vi "GetEdgeMenu.vi"(0 "reference":refnum<class "StateTransitionEdge.lvclass">, 5 "error in (no error)":errorcluster) -> (14 "reference out":refnum<class "StateTransitionEdge.lvclass">, 15 "MenuOptions":string[](array[string]), 19 "error out":errorcluster)   [LabVIEW 2016, in "StateTransitionEdge.lvclass"]
doc: "GetEdgeMenu"
uses:
  <resource>/Framework/Providers/Open_GDS/UML/StateTransitionEdge_class/StateTransitionEdge.lvclass
  C:/Program Files (x86)/National Instruments/LabVIEW 2016/resource/Framework/Providers/Open_GDS/UML/ClassRelationshipEdge_class/ClassRelationshipEdge.lvclass
  <resource>/Framework/Providers/Open_GDS/UML/ClassRelationshipEdge_class/ClassRelationshipEdge.lvclass
  <resource>/Framework/Providers/Open_GDS/UML/BentStyle_class/BentStyle.lvclass
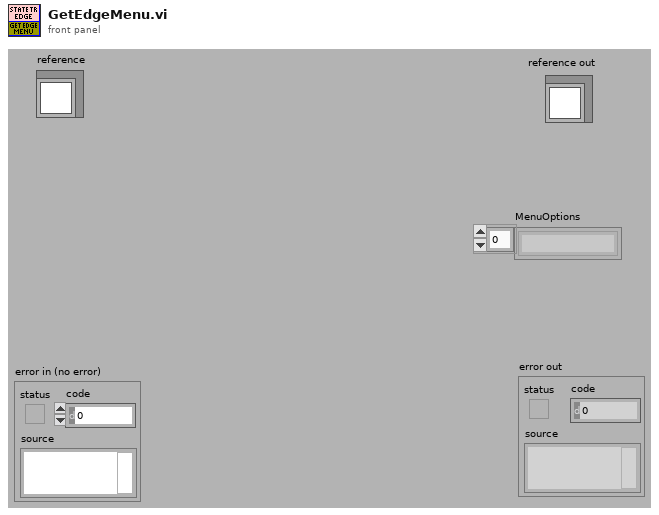
[diagram p1: front panel]
types:
  T1 = typedef "ClassRelationshipEdge.lvclass/ObjectAttributes.ctl" = cluster{"bentStyleRef":refnum<class "BentStyle.lvclass">, "startConnectionOffset":cluster{"x":i32, "y":i32}, "endConnectionOffset":cluster{"x":i32, "y":i32}, "MidLineOffset":cluster{"x":i32, "y":i32}, "DepClass":T2}
  T2 = typedef "ReversedEngineering_ViDependencyDetailsType.ctl" = cluster{"ThisVIs/Ctls":path[], "Dependent_VIs/Ctls":path[]}
  T3 = typedef "BentStyle.lvclass/BentStyleType.ctl" = enum16{"STRAIGHT", "HV", "VH", "HVH", "VHV", "ARC"}
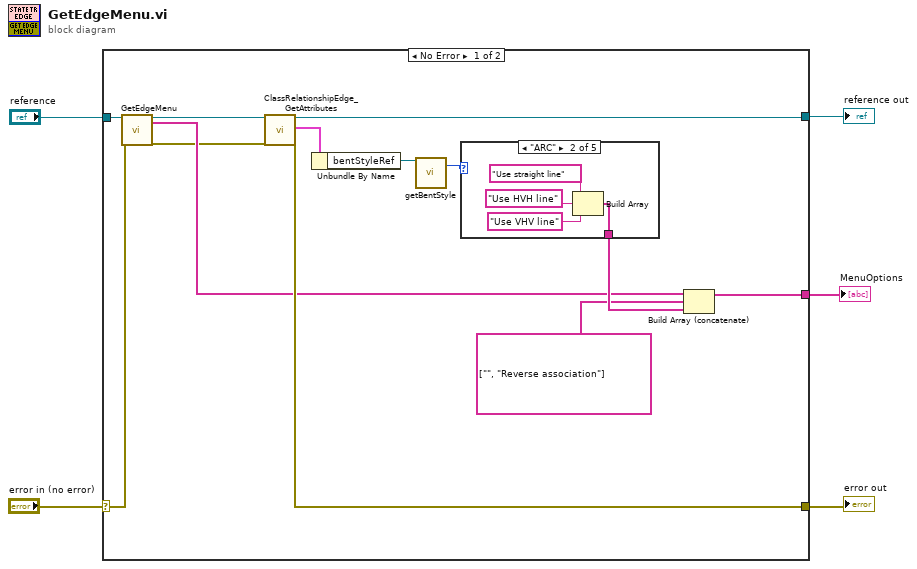
[diagram p0: block diagram]
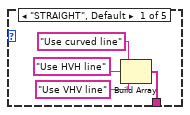
[diagram p2: hidden frame]
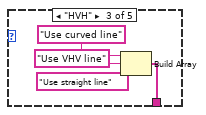
[diagram p3: hidden frame]
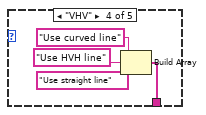
[diagram p4: hidden frame]
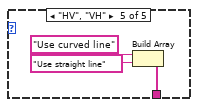
[diagram p5: hidden frame]
diagram:
  n1 = case shown="No Error" "error in (no error)" {
    selector: "error in (no error)" -> [w7 w38]
    tunnel: "reference" -> [w10 w39]
    tunnel: [w17 w38] -> w3
    tunnel: [w18 w39] -> w2
    tunnel: [w16 _] -> w1
    frame No Error {
      n2 = call-parent "GetEdgeMenu.vi"("reference"=w10, "error in (no error)"=w7) -> ("reference out"=w11:refnum<class "StateTransitionEdge.lvclass">, "MenuOptions"=w9:string[], "error out"=w8:errorcluster)  [unwired: 15 in]
      n3 = call <resource>:"ClassRelationshipEdge_GetAttributes.vi"("reference in"=w11, "error in (no error)"=w8) -> ("reference out"=w18:refnum<class "StateTransitionEdge.lvclass">, "Data"=w6:T1, "error out"=w17:errorcluster)  [unwired: 14 in, 1 out]
      n4 = Unbundle By Name(w6) -> ("bentStyleRef"=w15:refnum<class "BentStyle.lvclass">)
      n5 = call-dynamic "getBentStyle.vi"("reference"=w15) -> ("bentStyle"=w14:T3)  [unwired: 16 in, 2 out]
      n6 = case shown="\"ARC\"" w14 {
        tunnel: [w20 w24 w28 w32 w37] -> w13
        frame "STRAIGHT", Default {
          n7 = Build Array("Use curved line" ("String"), "Use HVH line" ("String"), "Use VHV line" ("String")) -> (w20:string[])
        }
        frame "ARC" {
          n8 = Build Array("Use straight line" ("String"), "Use HVH line" ("String"), "Use VHV line" ("String")) -> (w24:string[])
        }
        frame "HVH" {
          n9 = Build Array("Use curved line" ("String"), "Use VHV line" ("String"), "Use straight line" ("String")) -> (w28:string[])
        }
        frame "VHV" {
          n10 = Build Array("Use curved line" ("String"), "Use HVH line" ("String"), "Use straight line" ("String")) -> (w32:string[])
        }
        frame "HV", "VH" {
          n11 = Build Array("Use curved line" ("String"), "Use straight line" ("String")) -> (w37:string[])
        }
      }
      n12 = Build Array (concatenate)(w9, string[] ["", "Reverse association"] ("array"), w13) -> (w16:string[])
    }
    frame Error {
    }
  }
  "reference out" <- w2
  "error out" <- w3
  "MenuOptions" <- w1
